vi "SampleRotator main.vi"(9 "axis (0)":u32(ring) items=["1", "2", "3"], 10 "Top":refnum<queue>, 11 "Rotator":refnum<queue>) -> (3 "Ended":bool)   [LabVIEW 2024, in "SampleRotator.lvlib"]
doc: "This is a main VI of module for Sample rotator. It recives and executes commands, which comes from master controller. \nCommands and responses:\n\n/* */\nInitialize(path to driver DLL); -> Initialized(Contoller info<devN, devT, ID, Serial, Addr, connected?>);\n\n/* */\nUpdate(); -> Update(axis status<axis info, position, frequency, voltage>);\n\n/* */\nSetParameters(parameters<freq[Hz]; ampl[V]; offset[V]; tolerance[um]>); -> ParametersSet(parameters<freq; amp; offset; tolerance>);\n\n/* */\nSetPositon(positionToSet<relative?, double>) -> PositionSet(position to set<relative?, doubele);\n\n/* */\nEnd(), -> Disconnected();"
uses:
  SampleRotator.lvlib
  ctl/Rotator all.ctl
  ctl/Axis status.ctl
  Messenger service/Data types/Module name.ctl
  ctl/Motion Properties.ctl
  ctl/Positoin to set.ctl
  ctl/Rotator commands.ctl
panel:
  out "wrong capacity":bool
  out "Piezo\nstatus":T1 {"ActuatorType" items=["Linear", "Rotator", "Goniometer"]; "Features" format="%08b"; "FW-Version" format="%x"; "Controller info"."DeviceType" items=["ANC350res", "ANC350num", "ANC350fps", "No device / invalid"]; "Controller info"."ID" format="%x"}
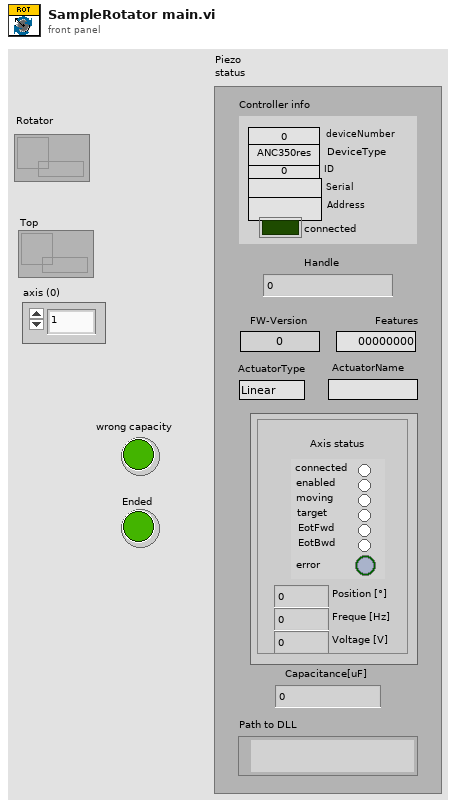
[diagram p1: front panel]
types:
  T1 = typedef "SampleRotator.lvlib/Rotator all.ctl" = cluster{"Controller info":cluster{"deviceNumber":i32, "DeviceType":i32, "ID":u32, "Serial":string, "Address":string, "connected":bool}, "Handle":u64, "FW-Version":i32, "Features":u32, "ActuatorType":u16, "ActuatorName":string, "Axis info":T2, "Capacitance[uF]":dbl, "Path to DLL":path}
  T2 = typedef "SampleRotator.lvlib/Axis status.ctl" = cluster{"Axis status":cluster{"connected":bool, "enabled":bool, "moving":bool, "target":bool, "EotFwd":bool, "EotBwd":bool, "error":bool}, "Position [°]":dbl, "Freque [Hz]":dbl, "Voltage [V]":dbl}
  T3 = typedef "SampleRotator.lvlib/Rotator commands.ctl" = enum16{"Ignore", "Initialize", "Update", "Set parameters", "Stop movement", "Set position", "Disconnect", "End"}
  T4 = typedef "Module name.ctl" = enum16{"Emty", "Magnet", "VTI", "Excitation", "Servo", "Acquisition", "Rotator", "Digitizer", "SMU2450", "Carousel", "Multimeter", "Tmp monitor", "Power monitor"}
  T5 = typedef "Motion Properties.ctl" = cluster{"Frequency [Hz]":dbl, "Precision [m°]":dbl, "DC voltage [V]":dbl, "Amplitude [V]":dbl}
  T6 = typedef "Positoin to set.ctl" = cluster{"Relative?":bool, "Position [°]":dbl, "Safe to move?":bool}
  T7 = cluster{"deviceNumber":i32, "DeviceType":i32, "ID":u32, "Serial":string, "Address":string, "connected":bool}
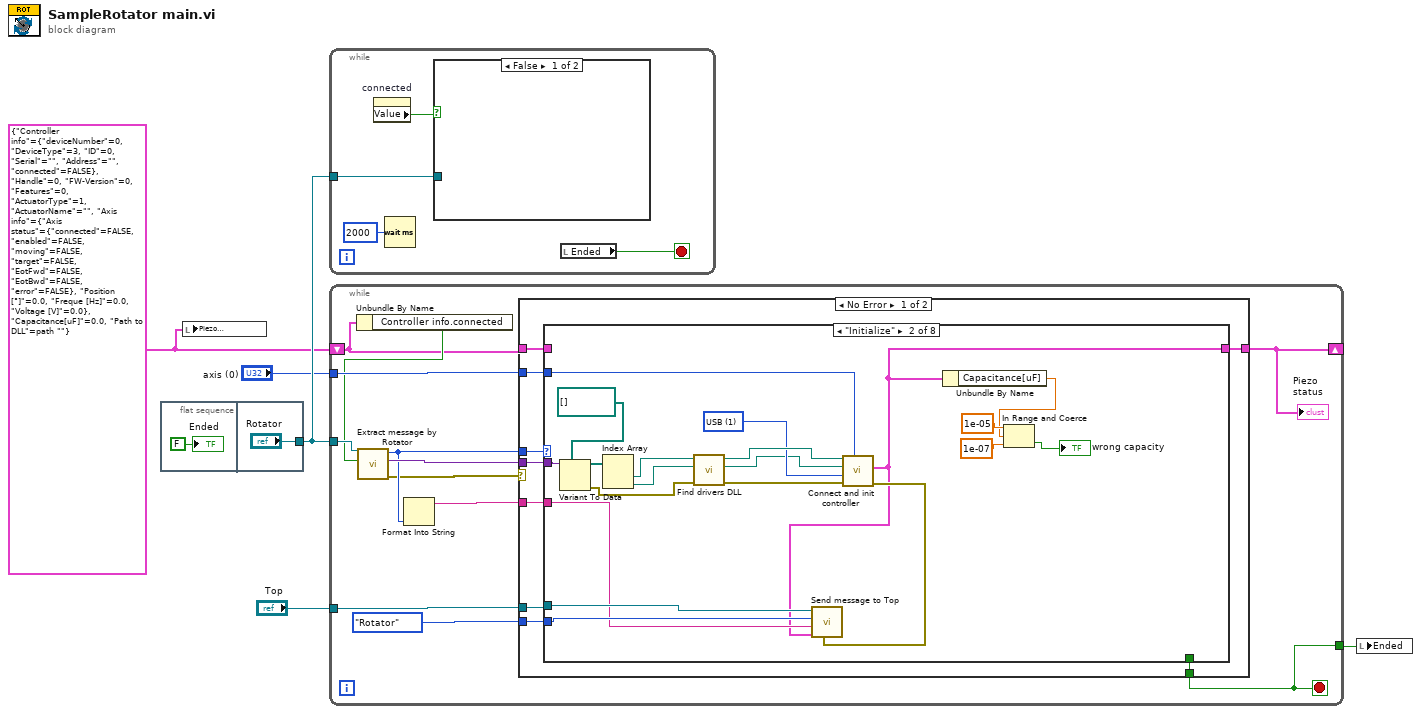
[diagram p0: block diagram]
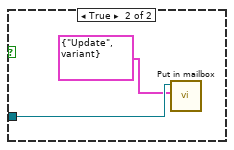
[diagram p2: hidden frame]
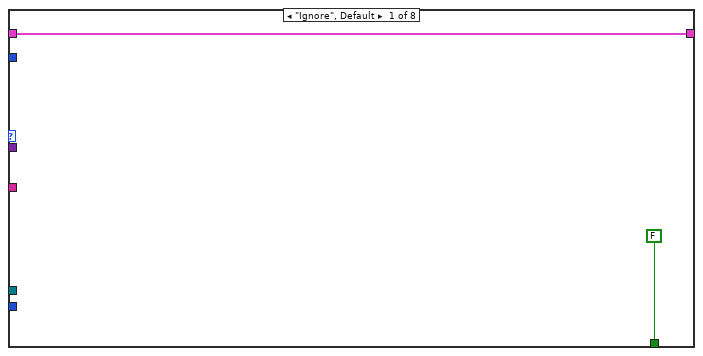
[diagram p3: hidden frame]
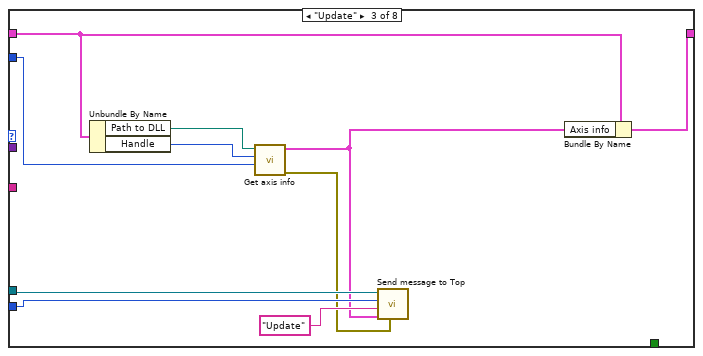
[diagram p4: hidden frame]
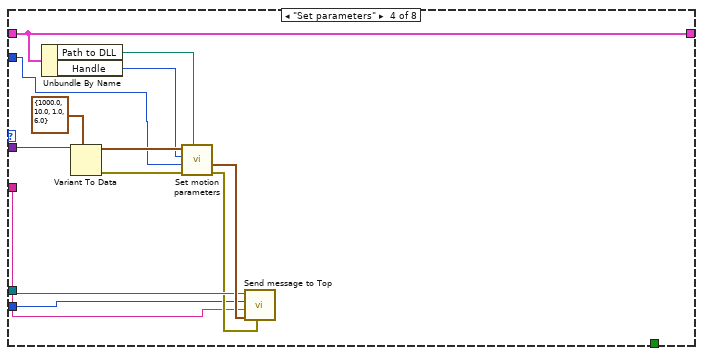
[diagram p5: hidden frame]
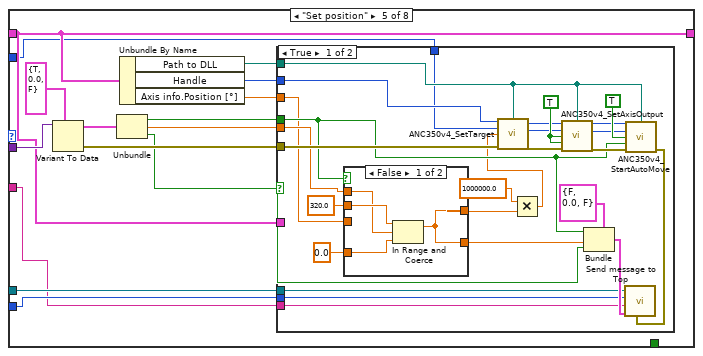
[diagram p6: hidden frame]
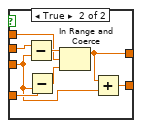
[diagram p7: hidden frame]
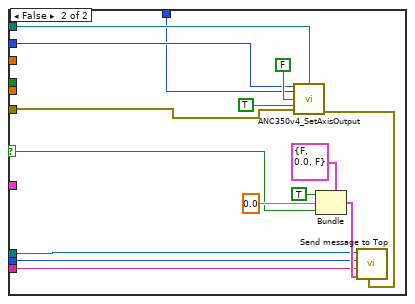
[diagram p8: hidden frame]
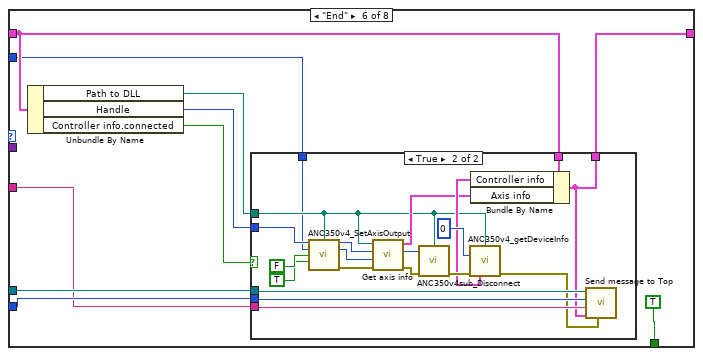
[diagram p9: hidden frame]
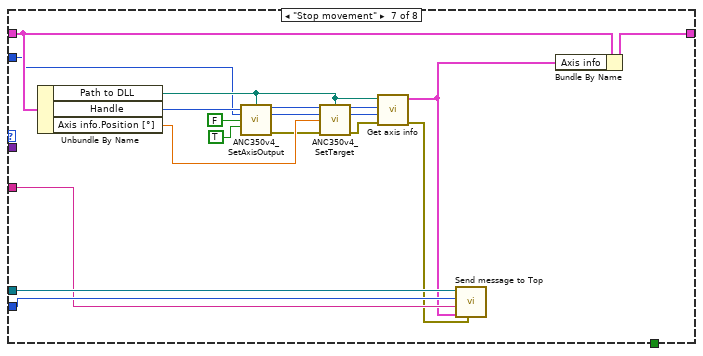
[diagram p11: hidden frame]
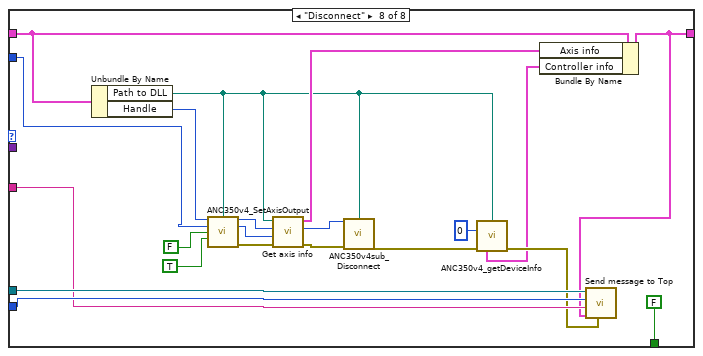
[diagram p12: hidden frame]
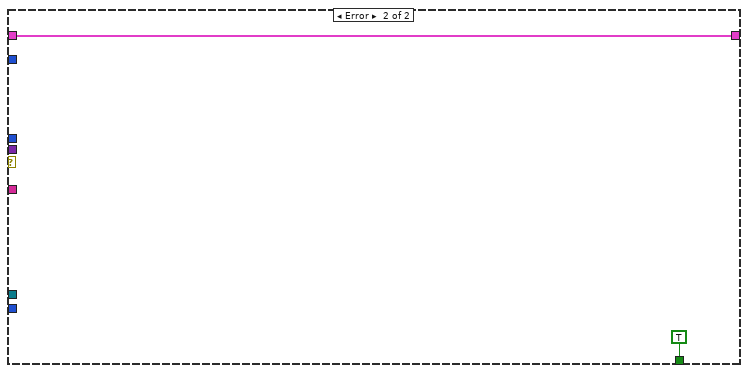
[diagram p13: hidden frame]
diagram:
  w2 = T1 {"Controller info"={"deviceNumber"=0, "DeviceType"=3, "ID"=0, "Serial"="", "Address"="", "connected"=FALSE}, "Handle"=0, "FW-Version"=0, "Features"=0, "ActuatorType"=1, "ActuatorName"="", "Axis info"={"Axis status"={"connected"=FALSE, "enabled"=FALSE, "moving"=FALSE, "target"=FALSE, "EotFwd"=FALSE, "EotBwd"=FALSE, "error"=FALSE}, "Position [°]"=0.0, "Freque [Hz]"=0.0, "Voltage [V]"=0.0}, "Capacitance[uF]"=0.0, "Path to DLL"=path ""} ("Rotator")
  n1 = flat-sequence {
    tunnel: ["Rotator"] -> w3
    frame #0 {
      "Ended" <- FALSE
    }
    frame #1 {
    }
  }
  n2 = local write "Piezo\nstatus"(w2) -> ()
  n3 = while {
    tunnel: w3 -> [w8]
    stop <- w10 stop-if-true
    n4 = property on="connected" class="Bool (strict)"() -> ("Value"=w9:bool)  [unwired: 2 in, 2 out]
    n5 = Wait (ms)(milliseconds to wait=u32 2000) -> ()  [unwired: 1 out]
    n6 = case shown="False" w9 {
      tunnel: w8 -> [_ w13]
      frame False {
      }
      frame True {
        n7 = call "Put in mailbox.vi"("Message"=cluster{"Command":T3, "Data":variant} {"Command"=enum."Update", "Data"=variant} ("MSG to rotator"), "Queue in"=w13) -> ()  [unwired: 7 in, 3 out]
      }
    }
    n8 = local read "Ended"() -> (w10:bool)
  }
  n9 = while {
    tunnel: "Top" -> [w25]
    shift-right: [w22] -> _
    shift-left: w2 -> [w14]
    tunnel: [w17] -> w4
    tunnel: w3 -> [w18]
    tunnel: "axis (0)" -> [w16]
    stop <- w17 stop-if-true
    n10 = Unbundle By Name(w14) -> ("Controller info.connected"=w15:bool)
    n11 = call "Extract message by Rotator.vi"("Initialized?"=w15, "Queue in"=w18) -> ("error out"=w19:errorcluster, "Data"=w23:variant, "Command out"=w21:T3)  [unwired: 6 in, 1 out]
    n12 = Format Into String(w21) -> (resulting string=w20:string)  [unwired: 3 in, 1 out]
    n13 = case shown="No Error" w19 {
      tunnel: w25 -> [w34 _]
      tunnel: Module_name."Rotator" ("Module name") -> [w33 _]
      tunnel: w23 -> [w32 _]
      tunnel: [w31 w221] -> w22
      tunnel: w14 -> [w30 w221]
      tunnel: [w29 TRUE] -> w17
      tunnel: w21 -> [w28 _]
      tunnel: w20 -> [w27 _]
      tunnel: w16 -> [w26 _]
      frame No Error {
        n14 = case shown="\"Initialize\"" w28 {
          tunnel: [FALSE _ _ _ _ TRUE _ FALSE] -> w29
          tunnel: w34 -> [_ w56 w66 w75 w87 w159 w199 w220]
          tunnel: w33 -> [_ w55 w65 w73 w88 w158 w198 w219]
          tunnel: w32 -> [_ w54 _ w77 w94 _ _ _]
          tunnel: [w35 w38 w59 w70 w92 w151 w193 w204] -> w31
          tunnel: w30 -> [w35 _ w60 w70 w92 w152 w196 w216]
          tunnel: w27 -> [_ w46 _ w72 w86 w156 w197 w217]
          tunnel: w26 -> [_ w37 w57 w67 w80 w150 w181 w200]
          frame "Ignore", Default {
          }
          frame "Initialize" {
            w45 = u32 1 items=["None", "USB", "TCP", "All"] ("Interface types")
            n15 = Variant To Data(type=path[] [], Variant=w54) -> (data=w52:path[], error out=w39:errorcluster)  [unwired: 1 in]
            n16 = Index Array(array=w52) -> (element #1=w43:path, element #2=w42:path)  [unwired: 2 in]
            n17 = call "Find drivers DLL.vi"("error in (no error)"=w39, "Path to LUT"=w42, "Path to DLL"=w43) -> ("error out"=w51:errorcluster, "LUT path out"=w44:path, "path out"=w47:path)  [unwired: 6 in]
            n18 = call "Connect and init controller.vi"("axis (0)"=w37, "error in (no error)"=w51, "Interface types"=w45, "path to LUT"=w44, "path to dll"=w47) -> ("error out"=w41:errorcluster, "Rotator"=w38:T1)  [unwired: 5 in]
            n19 = call "Send message to Top.vi"("Error in (no error)"=w41, "Data"=w38, "Response"=w46, "Module"=w55, "Mailbox address in"=w56) -> ()  [unwired: 5 in, 2 out]
            n20 = Unbundle By Name(w38) -> ("Capacitance[uF]"=w40:dbl)
            n21 = In Range and Coerce(upper limit=1e-05, x=w40, lower limit=1e-07) -> (In Range?=→"wrong capacity":bool)  [unwired: 1 out]
          }
          frame "Update" {
            n22 = Unbundle By Name(w60) -> ("Path to DLL"=w62:path, "Handle"=w61:u64)
            n23 = call "Get axis info.vi"("axis"=w57, "deviceHandle"=w61, "path in"=w62) -> ("error out"=w63:errorcluster, "Axis status"=w58:T2)  [unwired: 5 in, 2 out]
            n24 = call "Send message to Top.vi"("Error in (no error)"=w63, "Data"=w58, "Response"="Update", "Module"=w65, "Mailbox address in"=w66) -> ()  [unwired: 5 in, 2 out]
            n25 = Bundle By Name(cluster=w60, "Axis info"=w58) -> (w59:T1)
          }
          frame "Set parameters" {
            n26 = Unbundle By Name(w70) -> ("Path to DLL"=w68:path, "Handle"=w69:u64)
            n27 = Variant To Data(type=T5 {"Frequency [Hz]"=1000.0, "Precision [m°]"=10.0, "DC voltage [V]"=1.0, "Amplitude [V]"=6.0} ("Motion parameters"), Variant=w77) -> (data=w79:T5, error out=w78:errorcluster)  [unwired: 1 in]
            n28 = call "Set motion parameters.vi"("path in"=w68, "error in (no error)"=w78, "axis in"=w67, "deviceHandle in"=w69, "Motion parameters"=w79) -> ("error out"=w74:errorcluster, "Motion parameters out"=w76:T5)  [unwired: 3 in, 2 out]
            n29 = call "Send message to Top.vi"("Error in (no error)"=w74, "Data"=w76, "Response"=w72, "Module"=w73, "Mailbox address in"=w75) -> ()  [unwired: 5 in, 2 out]
          }
          frame "Set position" {
            n30 = Variant To Data(type=T6 {"Relative?"=TRUE, "Position [°]"=0.0, "Safe to move?"=FALSE}, Variant=w94) -> (data=w91:T6, error out=w90:errorcluster)  [unwired: 1 in]
            n31 = Unbundle(w91) -> ("Relative?"=w89:bool, "Position [°]"=w85:dbl, "Safe to move?"=w84:bool)
            n32 = Unbundle By Name(w92) -> ("Path to DLL"=w81:path, "Handle"=w82:u64, "Axis info.Position [°]"=w83:dbl)
            n33 = case shown="True" w84 {
              selector: w84 -> [w99 w139]
              tunnel: w92 -> [_ _]
              tunnel: w90 -> [w114 w140]
              tunnel: w89 -> [w110 _]
              tunnel: w88 -> [w107 w145]
              tunnel: w87 -> [w106 w144]
              tunnel: w86 -> [w104 w143]
              tunnel: w85 -> [w102 _]
              tunnel: w83 -> [w98 _]
              tunnel: w82 -> [w97 w136]
              tunnel: w81 -> [w96 w138]
              tunnel: w80 -> [w95 w135]
              frame True {
                w121 = TRUE ("autoDisable")
                n34 = case shown="False" w110 {
                  tunnel: w102 -> [w124 w130]
                  tunnel: w98 -> [_ w129]
                  tunnel: [w123 w127] -> w109
                  tunnel: 320.0 ("lower limit") -> [w126 w132]
                  tunnel: 0.0 ("upper limit") -> [w125 w131]
                  tunnel: [w123 w128] -> w103
                  frame False {
                    n35 = In Range and Coerce(upper limit=w126, x=w124, lower limit=w125) -> (coerced(x)=w123:dbl)  [unwired: 1 out]
                  }
                  frame True {
                    n36 = Subtract(x=w132, y=w129) -> (x-y=w134:dbl)
                    n37 = Subtract(x=w131, y=w129) -> (x-y=w133:dbl)
                    n38 = In Range and Coerce(upper limit=w134, x=w130, lower limit=w133) -> (coerced(x)=w127:dbl)  [unwired: 1 out]
                    n39 = Add(x=w127, y=w129) -> (x+y=w128:dbl)
                  }
                }
                n40 = Multiply(x=1000000.0, y=w109) -> (x*y=w101:dbl)
                n41 = call <instrlib>:"ANC350v4_SetTarget.vi"("deviceHandle"=w97, "Path to *.DLL"=w96, "axis"=w95, "Target [µm | m°]"=w101, "error in"=w114) -> ("deviceHandle"=w116:u64, "axis"=w115:u8, "error ANC350v4_setTarget"=w120:errorcluster)  [unwired: 8 in]
                n42 = call <instrlib>:"ANC350v4_SetAxisOutput.vi"("deviceHandle"=w116, "Path to *.DLL"=w96, "axis"=w115, "enable"=w121, "autoDisable"=w121, "error in"=w120) -> ("deviceHandle"=w118:u64, "axis"=w117:u8, "error ANC350v4_setAxisOutput"=w119:errorcluster)  [unwired: 7 in]
                n43 = Bundle(cluster=T6 {"Relative?"=FALSE, "Position [°]"=0.0, "Safe to move?"=FALSE}, "Relative?"=w110, "Position [°]"=w103, "Safe to move?"=w99) -> (w108:T6)
                n44 = call <instrlib>:"ANC350v4_StartAutoMove.vi"("deviceHandle"=w118, "Path to *.DLL"=w96, "axis"=w117, "Enable | Disable"=TRUE, "Relative | Absolute"=w110, "error in"=w119) -> ("error ANC350v4_StartAutoMove"=w105:errorcluster)  [unwired: 7 in, 2 out]
                n45 = call "Send message to Top.vi"("Error in (no error)"=w105, "Data"=w108, "Response"=w104, "Module"=w107, "Mailbox address in"=w106) -> ()  [unwired: 5 in, 2 out]
              }
              frame False {
                n46 = call <instrlib>:"ANC350v4_SetAxisOutput.vi"("deviceHandle"=w136, "Path to *.DLL"=w138, "axis"=w135, "enable"=FALSE ("autoDisable"), "autoDisable"=TRUE, "error in"=w140) -> ("error ANC350v4_setAxisOutput"=w148:errorcluster)  [unwired: 7 in, 2 out]
                n47 = Bundle(cluster=T6 {"Relative?"=FALSE, "Position [°]"=0.0, "Safe to move?"=FALSE}, "Relative?"=TRUE, "Position [°]"=0.0, "Safe to move?"=w139) -> (w146:T6)
                n48 = call "Send message to Top.vi"("Error in (no error)"=w148, "Data"=w146, "Response"=w143, "Module"=w145, "Mailbox address in"=w144) -> ()  [unwired: 5 in, 2 out]
              }
            }
          }
          frame "End" {
            n49 = Unbundle By Name(w152) -> ("Path to DLL"=w155:path, "Handle"=w154:u64, "Controller info.connected"=w153:bool)
            n50 = case shown="True" w153 {
              tunnel: w159 -> [_ w180]
              tunnel: w158 -> [_ w179]
              tunnel: w156 -> [_ w178]
              tunnel: w155 -> [_ w164]
              tunnel: w154 -> [_ w177]
              tunnel: w152 -> [w160 w173]
              tunnel: [w160 w163] -> w151
              tunnel: w150 -> [_ w161]
              frame False {
              }
              frame True {
                n51 = call <instrlib>:"ANC350v4_SetAxisOutput.vi"("deviceHandle"=w177, "Path to *.DLL"=w164, "axis"=w161, "enable"=FALSE, "autoDisable"=TRUE) -> ("deviceHandle"=w165:u64, "axis"=w166:u8, "error ANC350v4_setAxisOutput"=w170:errorcluster)  [unwired: 8 in]
                n52 = call "Get axis info.vi"("error in"=w170, "axis"=w166, "deviceHandle"=w165, "path in"=w164) -> ("error out"=w169:errorcluster, "deviceHandle out"=w167:u64, "Axis status"=w168:T2)  [unwired: 4 in, 1 out]
                n53 = call <instrlib>:"ANC350v4sub_Disconnect.vi"("ANC350v4_Handle"=w167, "Path to *.DLL"=w164, "error in"=w169) -> ("error ANC350v4_Dis/Connect"=w176:errorcluster)  [unwired: 12 in]
                n54 = call <instrlib>:"ANC350v4_getDeviceInfo.vi"("Path to *.DLL"=w164, "deviceNumber"=u32 0, "error in"=w176) -> ("output cluster"=w172:T7, "Error_ANC350v4_getDeviceInfo"=w175:errorcluster)  [unwired: 5 in, 6 out]
                n55 = Bundle By Name(cluster=w173, "Controller info"=w172, "Axis info"=w168) -> (w163:T1)
                n56 = call "Send message to Top.vi"("Error in (no error)"=w175, "Data"=w163, "Response"=w178, "Module"=w179, "Mailbox address in"=w180) -> ()  [unwired: 5 in, 2 out]
              }
            }
          }
          frame "Stop movement" {
            n57 = Unbundle By Name(w196) -> ("Path to DLL"=w186:path, "Handle"=w195:u64, "Axis info.Position [°]"=w189:dbl)
            n58 = call <instrlib>:"ANC350v4_SetAxisOutput.vi"("deviceHandle"=w195, "Path to *.DLL"=w186, "axis"=w181, "enable"=FALSE, "autoDisable"=TRUE) -> ("deviceHandle"=w188:u64, "axis"=w187:u8, "error ANC350v4_setAxisOutput"=w182:errorcluster)  [unwired: 8 in]
            n59 = call <instrlib>:"ANC350v4_SetTarget.vi"("deviceHandle"=w188, "Path to *.DLL"=w186, "axis"=w187, "Target [µm | m°]"=w189, "error in"=w182) -> ("deviceHandle"=w185:u64, "axis"=w184:u8, "error ANC350v4_setTarget"=w183:errorcluster)  [unwired: 8 in]
            n60 = call "Get axis info.vi"("error in"=w183, "axis"=w184, "deviceHandle"=w185, "path in"=w186) -> ("error out"=w194:errorcluster, "Axis status"=w192:T2)  [unwired: 4 in, 2 out]
            n61 = call "Send message to Top.vi"("Error in (no error)"=w194, "Data"=w192, "Response"=w197, "Module"=w198, "Mailbox address in"=w199) -> ()  [unwired: 5 in, 2 out]
            n62 = Bundle By Name(cluster=w196, "Axis info"=w192) -> (w193:T1)
          }
          frame "Disconnect" {
            n63 = Unbundle By Name(w216) -> ("Path to DLL"=w202:path, "Handle"=w215:u64)
            n64 = call <instrlib>:"ANC350v4_SetAxisOutput.vi"("deviceHandle"=w215, "Path to *.DLL"=w202, "axis"=w200, "enable"=FALSE, "autoDisable"=TRUE) -> ("deviceHandle"=w213:u64, "axis"=w212:u8, "error ANC350v4_setAxisOutput"=w211:errorcluster)  [unwired: 8 in]
            n65 = call "Get axis info.vi"("error in"=w211, "axis"=w212, "deviceHandle"=w213, "path in"=w202) -> ("error out"=w208:errorcluster, "deviceHandle out"=w210:u64, "Axis status"=w209:T2)  [unwired: 4 in, 1 out]
            n66 = call <instrlib>:"ANC350v4sub_Disconnect.vi"("ANC350v4_Handle"=w210, "Path to *.DLL"=w202, "error in"=w208) -> ("error ANC350v4_Dis/Connect"=w207:errorcluster)  [unwired: 12 in]
            n67 = call <instrlib>:"ANC350v4_getDeviceInfo.vi"("Path to *.DLL"=w202, "deviceNumber"=u32 0, "error in"=w207) -> ("output cluster"=w203:T7, "Error_ANC350v4_getDeviceInfo"=w205:errorcluster)  [unwired: 5 in, 6 out]
            n68 = Bundle By Name(cluster=w216, "Axis info"=w209, "Controller info"=w203) -> (w204:T1)
            n69 = call "Send message to Top.vi"("Error in (no error)"=w205, "Data"=w204, "Response"=w217, "Module"=w219, "Mailbox address in"=w220) -> ()  [unwired: 5 in, 2 out]
          }
        }
      }
      frame Error {
      }
    }
    "Piezo\nstatus" <- w22
  }
  n70 = local write "Ended"(w4) -> ()
